vi "Set BC.vi"(8 "error in (no error)":errorcluster, 10 "BC":variant, 11 "BC_Evolut_1D_VIRef in":refnum<class "NI_BC_Evolut_1D_VIRef.lvclass">) -> (0 "error out":errorcluster, 3 "BC_Evolut_1D_VIRef out":refnum<class "NI_BC_Evolut_1D_VIRef.lvclass">)   [LabVIEW 2020, in "NI_PDE.lvlib" / "NI_BC_Evolut_1D_VIRef.lvclass"]
uses:
  <vilib>/gmath/pde.llb/BCClass/BC_Evolut_1D_VIRef/NI_BC_Evolut_1D_VIRef.lvclass
  <vilib>/gmath/pde.llb/BCClass/BC_Evolut_1D_VIRef/BC Data.ctl
  <vilib>/gmath/pde.llb/Common/PDE_BC Type.ctl
  <vilib>/gmath/pde.llb/Common/PDE_BC Position 1D.ctl
  <vilib>/gmath/pde.llb/BCClass/BC_Evolut_1D_VIRef/NI_BC_Evolut_1D_VIRef.lvclass/NI_BC_Evolut_1D_VIRef.ctl
  <vilib>/gmath/NI_PDE.lvlib
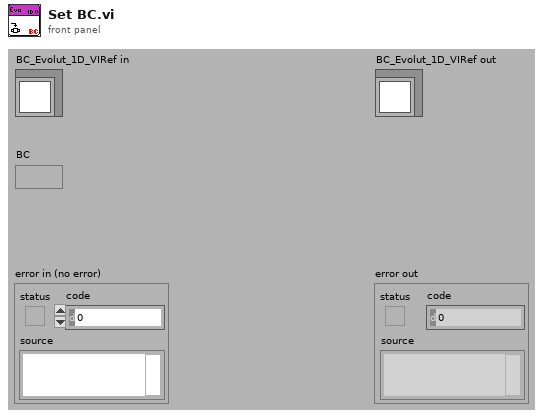
[diagram p1: front panel]
types:
  T1 = typedef "NI_PDE.lvlib/NI_BC_Evolut_1D_VIRef.lvclass/BC Data.ctl" = cluster{"type":T2, "position":T3, "G":refnum<vi>, "data":variant}
  T2 = typedef "NI_PDE.lvlib/PDE_BC Type.ctl" = i32
  T3 = typedef "NI_PDE.lvlib/PDE_BC Position 1D.ctl" = i32
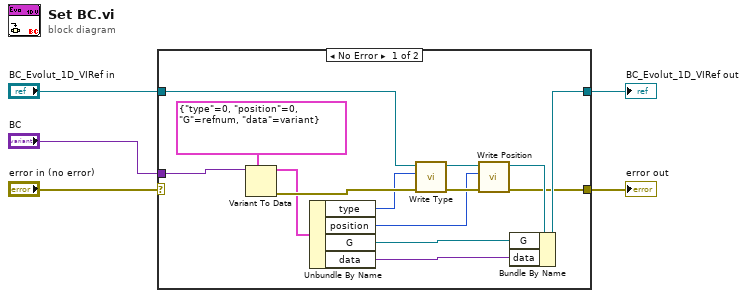
[diagram p0: block diagram]
diagram:
  n1 = case shown="No Error" "error in (no error)" {
    selector: "error in (no error)" -> [_ w21]
    tunnel: "BC_Evolut_1D_VIRef in" -> [w16 w20]
    tunnel: [w9 w20] -> w5
    tunnel: [w8 w21] -> w4
    tunnel: "BC" -> [w11 _]
    frame No Error {
      n2 = Variant To Data(type=T1 {"type"=0, "position"=0, "G"=refnum, "data"=variant} ("BC data"), Variant=w11) -> (data=w14:T1, error out=w15:errorcluster)  [unwired: 1 in]
      n3 = Unbundle By Name(w14) -> ("type"=w13:T2, "position"=w12:T3, "G"=w7:refnum<vi>, "data"=w6:variant)
      n4 = call-dynamic "Write Type.vi"("error in (no error)"=w15, "BC type"=w13, "BC.lvclass in"=w16) -> ("error out"=w17:errorcluster, "BC.lvclass out"=w18:refnum<class "NI_BC_Evolut_1D_VIRef.lvclass">)  [unwired: 7 out]
      n5 = call-dynamic "Write Position.vi"("error in (no error)"=w17, "BC position 1D"=w12, "BC_Evolut_1D.lvclass in"=w18) -> ("error out"=w8:errorcluster, "BC_Evolut_1D.lvclass out"=w10:refnum<class "NI_BC_Evolut_1D_VIRef.lvclass">)  [unwired: 7 out]
      n6 = Bundle By Name(cluster=w10, "G"=w7, "data"=w6) -> (w9:refnum<class "NI_BC_Evolut_1D_VIRef.lvclass">)
    }
    frame Error {
    }
  }
  "BC_Evolut_1D_VIRef out" <- w5
  "error out" <- w4
